vi "Move LPSTR to String.vi"(0 "LPSTR":u64) -> (2 "String":string)   [LabVIEW 2013, in "libssh2.lvlib"]
uses:
  libssh2.lvlib
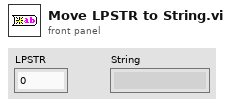
[diagram p1: front panel]
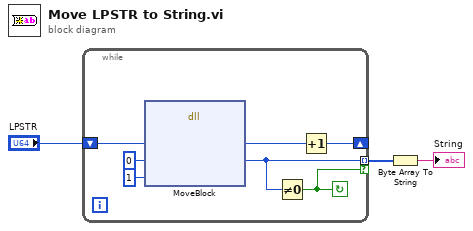
[diagram p0: block diagram]
diagram:
  n1 = while {
    tunnel: [w7] -> w3 mode=indexing if=w4
    shift-right: [w5] -> _
    shift-left: "LPSTR" -> [w10]
    stop <- w4 continue-if-true
    n2 = dll-call lib="LabVIEW" fn="MoveBlock"("ps"=w10, "pd"=u8 0, "size"=u32 1) -> ("ps"=w6:u64, "pd"=w7:u8)  [unwired: 5 in, 2 out]
    n3 = Not Equal To 0?(x=w7) -> (x != 0?=w4:bool)
    n4 = Increment(x=w6) -> (x+1=w5:u64)
  }
  n5 = Byte Array To String(unsigned byte array=w3) -> (string=→"String":string)
